vi "Robot Kalman Filter And Update.vi"(10 "Cluster in":T3 {"Detection Robot"."height" format="%+4.3f"; "Detection Robot"."pixel_y" format="%+4.3f"; "Detection Robot"."pixel_x" format="%+4.3f"; "Detection Robot"."orientation" format="%+4.3f"; "Detection Robot"."y" format="%+4.3f"; "Detection Robot"."confidence" format="%4.3f"; "Detection Robot"."x" format="%+4.3f"}, 11 "Detection Robot":T1 {"height" format="%+4.3f"; "pixel_y" format="%+4.3f"; "pixel_x" format="%+4.3f"; "orientation" format="%+4.3f"; "y" format="%+4.3f"; "confidence" format="%4.3f"; "x" format="%+4.3f"}) -> (3 "Cluster out":T4 {"Detection Robot out"."height" format="%+4.3f"; "Detection Robot out"."pixel_y" format="%+4.3f"; "Detection Robot out"."pixel_x" format="%+4.3f"; "Detection Robot out"."orientation" format="%+4.3f"; "Detection Robot out"."y" format="%+4.3f"; "Detection Robot out"."confidence" format="%4.3f"; "Detection Robot out"."x" format="%+4.3f"})   [LabVIEW 2016]
uses:
  SSL Detection Robot.ctl
  <vilib>/Analysis/Matrix/Datatypes/RealMatrix.ctl
  Get Robot Pose.vi
  <vilib>/Analysis/Matrix/Numeric/Conversions/Array To Matrix - RA.vi
  <vilib>/Analysis/Matrix/NI_Matrix.lvlib
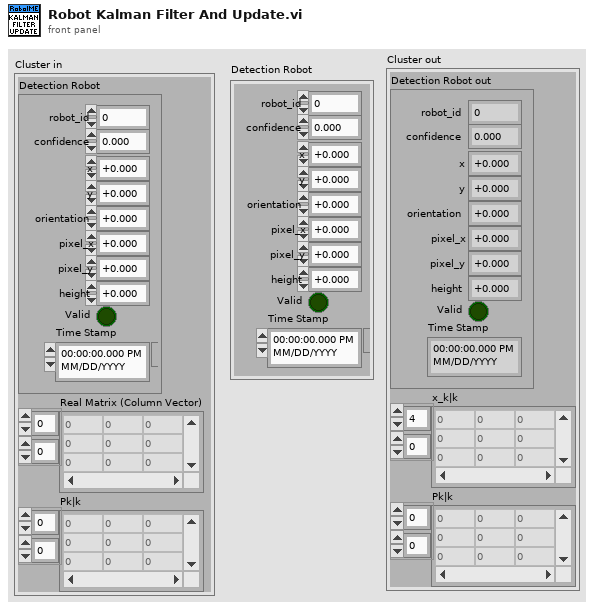
[diagram p1: front panel]
types:
  T1 = typedef "SSL Detection Robot.ctl" = cluster{"x":sgl, "robot_id":u32, "confidence":sgl, "y":sgl, "orientation":sgl, "pixel_x":sgl, "pixel_y":sgl, "height":sgl, "Valid":bool, "Time Stamp":timestamp}
  T2 = typedef "NI_Matrix.lvlib/RealMatrix.ctl" = dbl[][]
  T3 = cluster{"Detection Robot":T1, "Real Matrix (Column Vector)":T2, "Pk|k":T2}
  T4 = cluster{"Detection Robot out":T1, "x_k|k":T2, "Pk|k":T2}
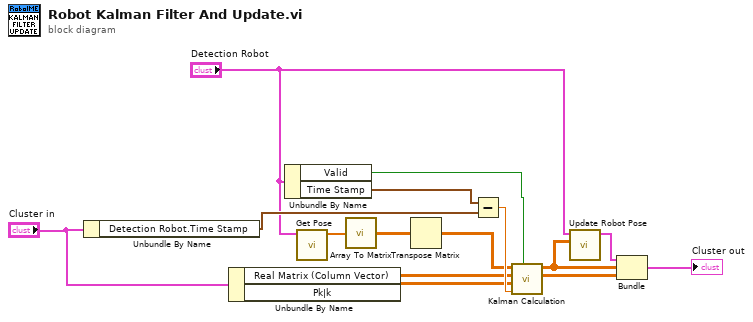
[diagram p0: block diagram]
diagram:
  n1 = Unbundle By Name("Cluster in") -> ("Detection Robot.Time Stamp"=w14:timestamp)
  n2 = Unbundle By Name("Cluster in") -> ("Real Matrix (Column Vector)"=w9:T2, "Pk|k"=w10:T2)
  n3 = Unbundle By Name("Detection Robot") -> ("Valid"=w12:bool, "Time Stamp"=w13:timestamp)
  n4 = call-poly "Get Pose.vi"("Detection Robot"="Detection Robot") -> ("Pose"=w4:sgl[])  [unwired: 10 in]
  n5 = call-poly <vilib>:"Array To Matrix.vi"("Real 1D Array"=w4) -> ("Real Matrix (Column Vector)"=w6:T2)
  n6 = Transpose Matrix(1:w6) -> (0:w5:T2)
  n7 = Subtract(x=w13, y=w14) -> (x-y=w15:dbl)
  n8 = call "Kalman Calculation.vi"("Use Observation"=w12, "iteração"=w15, "Pk-1|k-1"=w10, "x_k-1|k-1"=w9, "z_k"=w5) -> ("Pk|k"=w8:T2, "x_k|k"=w7:T2)  [unwired: 4 in, 1 out]
  n9 = call "Update Robot Pose.vi"("x_k|k"=w7, "Detection Robot in"="Detection Robot") -> ("Detection Robot out"=w11:T1)  [unwired: 9 in]
  n10 = Bundle("Detection Robot out"=w11, "x_k|k"=w7, "Pk|k"=w8) -> (→"Cluster out":T4)  [unwired: 1 in]
